vi "sub_KeyString.vi"(10 "String":string) -> (2 "Key String":string)   [LabVIEW 2014]
doc: "------------------------------------\nAuther: Koji Ohashi\nCopyright (c) 2020 Japan LabVIEW Users Group, Volunteer members.\nThis VI is released under the MIT License.\nhttp://opensource.org/licenses/mit-license.php\n------------------------------------"
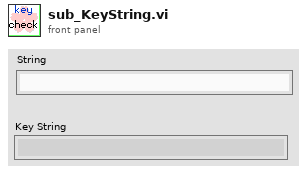
[diagram p1: front panel]
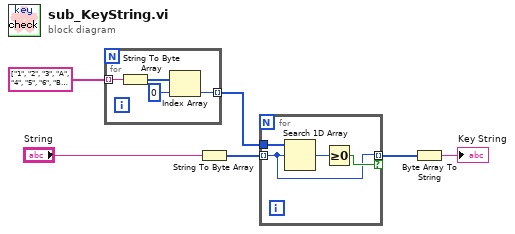
[diagram p0: block diagram]
diagram:
  n1 = for {
    tunnel: string[] ["1", "2", "3", "A", "4", "5", "6", "B", "7", "8", "9", "C", "*", "0", "#", "D"] ("1D array") -> [w10] mode=indexing
    tunnel: [w7] -> w4 mode=indexing
    n2 = String To Byte Array(string=w10) -> (unsigned byte array=w9:u8[])
    n3 = Index Array(array=w9, index=0) -> (element=w7:u8)
  }
  n4 = String To Byte Array(string="String") -> (unsigned byte array=w3:u8[])
  n5 = for {
    tunnel: w4 -> [w14]
    tunnel: w3 -> [w11] mode=indexing
    tunnel: [w11] -> w2 mode=indexing if=w12
    n6 = Search 1D Array(1D array=w14, element=w11) -> (index of element=w13:i32)  [unwired: 1 in]
    n7 = Greater Or Equal To 0?(x=w13) -> (x >= 0?=w12:bool)
  }
  n8 = Byte Array To String(unsigned byte array=w2) -> (string=→"Key String":string)
